vi "mhk_Basic Acquisition_XLS dbl.vi"() -> ()   [LabVIEW 2010]
uses:
  <vilib>/Utility/error.llb/DialogType.ctl
  <vilib>/DAQmx/read.llb/DAQmx Read (Analog 2D DBL NChan NSamp).vi
  <vilib>/DAQmx/create/channels.llb/DAQmx Create Channel (AI-Voltage-Basic).vi
  <vilib>/DAQmx/configure/timing.llb/DAQmx Timing (Sample Clock).vi
  <vilib>/daqmx/miscellaneous.llb/DAQmx Fill In Error Info.vi
  <vilib>/Utility/file.llb/Write To Spreadsheet File (DBL).vi
panel:
  out "# of pts per \nchannel":i32=100
  out "# of channels \nacquired":i32=2
  out "dt (sec)":dbl=0.0001
  in  "Save Data?":bool caption="Enable"
  in  "Maximum Value":dbl=5.0 format="%0.2f"
  in  "Minimum Value":dbl=-5.0 format="%0.2f"
  in  "Physical Channel":tag="Dev2/ai1:2"
  in  "Rate":dbl=10000.0 caption="Sample Rate (Hz)" format="%0.2f"
  in  "Samples per Channel":i32=100
  out "Measurement":cluster{i32, dbl, dbl[][]}(graph)={0, 0.0001, [[0.11978514969328898, 0.31235694448683127, 0.5038605914487136, 0.9799493392742699, 1.3254188665425581, 1.5303506576738792, 1.7484054078798792, 1.9394512771996215, 2.446058534501175, 2.4918362987151705, 2.93603320413831, 2.975402081362346, 3.4054078798791467, 3.576158940397351, 3.8329721976378672, 3.956266975920896, 4.169743949705496, 4.3510238959929195, 4.386120181890316, 4.5689260536515395, 4.546189764091921, 4.728995635853145, 4.6163823358867155, 4.819635608996856, 4.770348216193121, 4.813226722006897, 4.697256385998108, 4.821619312112796, 4.775994140446181, 4.627063814203314, 4.619434186834315, 4.470046082949309, 4.2544328135013885, 4.333475753044222, 4.042023987548448, 3.902401806695761, 3.7987914670247505, 3.4376049073763237, 3.230994598223823, 2.945036164433729, 2.93557542649617, 2.576525162511063, 2.383648182622761, 1.945860164189581, 1.641285439619129, 1.5956602679525131, 1.1384929960020753, 0.9956663716544084, 0.5467390972624897, 0.21317178868984038, 0.07248146000549333, -0.3666798913541063, -0.47242652668843654, -0.8313241981261635, -1.2146366771446881, -1.4604632709738457, -1.717886898403882, -2.0393993957335126, -2.228156376842555, -2.4820703756828517, -2.903378398998993, -3.0289620654927214, -3.4209723197119053, -3.6365855891598255, -3.7022003845332194, -3.8224433118686485, -3.945432905056917, -4.382610553300577, -4.406109805597095, -4.446699423200171, -4.618823816644795, -4.586626789147618, -4.89638966032899, -4.943693350016785, -4.701528977324747, -4.8908963286233105, -4.927671132541887, -4.89410077211829, -4.78408154545732, -4.791405987731559, -4.520554216132084, -4.551377910702842, -4.387188329721976, -4.12991729483932, -4.166997283852656, -3.988616595965453, -3.872493667409284, -3.493301187170019, -3.347880489516892, -2.953886532181768, -2.865840632343516, -2.6267281105990783, -2.461012604144414, -2.0392468031861326, -1.7902157658619953, -1.358073671681875, -1.259956663716544, -0.9611804559465316, -0.511490218817713, -0.3338724936674093], [0.48097170934171574, 0.5813776055177465, 1.0701315347758416, 1.3006988738670002, 1.4848780785546434, 2.024445326090274, 2.28354747154149, 2.377391888180181, 2.8096865749076816, 2.9644154179509874, 3.224433118686483, 3.325296792504654, 3.5700552385021513, 3.7896359141819516, 4.040955839716788, 4.079561754203925, 4.179204687643056, 4.556108279671621, 4.571520126956999, 4.757835627307962, 4.866023743400373, 4.8271126438184755, 4.6812341685232095, 4.770653401287881, 4.831080050050356, 4.752342295602283, 4.935148167363506, 4.6653645435956905, 4.738151188695944, 4.67909787285989, 4.609515671254616, 4.408398693807794, 4.144108401745659, 3.903012176885281, 3.9382610553300577, 3.80230109561449, 3.4612567522202218, 3.3538315988647116, 3.0941190832239753, 2.641224402600177, 2.359080782494583, 2.3191015350810265, 1.8089846491897337, 1.8016602069154943, 1.5018158513138218, 1.2016663106173895, 0.8290353099154637, 0.46800134281441697, 0.12222663045136875, -0.18448438978240303, -0.4924161503952147, -0.6015198217719047, -0.967589342936491, -1.2805566576128422, -1.4664143803216652, -1.7743461409344767, -2.0285653248695334, -2.414471877193518, -2.7007354960783716, -3.0053102206488234, -3.108157597582934, -3.392590105899228, -3.595843379009369, -3.7598803674428543, -3.9182714316232796, -4.154942472609638, -4.303567613757744, -4.400311288796655, -4.573656422620319, -4.791100802636799, -4.645527512436293, -4.832453382976776, -4.792474135563219, -4.920041505172887, -4.7949156163212985, -4.916684469130527, -4.857020783104953, -4.829096346934416, -4.718619342631306, -4.5365764336069825, -4.4392223883785515, -4.475081637012848, -4.183019501327555, -3.9310892056031985, -3.783989989928892, -3.6460463270973844, -3.3169042023987547, -3.087710196234016, -3.055207983642079, -2.687002166814173, -2.5399029511398665, -2.2985015411847285, -1.9431134983367413, -1.6838587603381452, -1.2489700003051851, -1.173741874446852, -0.7335123752555925, -0.5098117007965332, -0.06988738670003357, -0.02075258644367809]]}
  # "Channel Parameters"
  # "Timing Parameters"
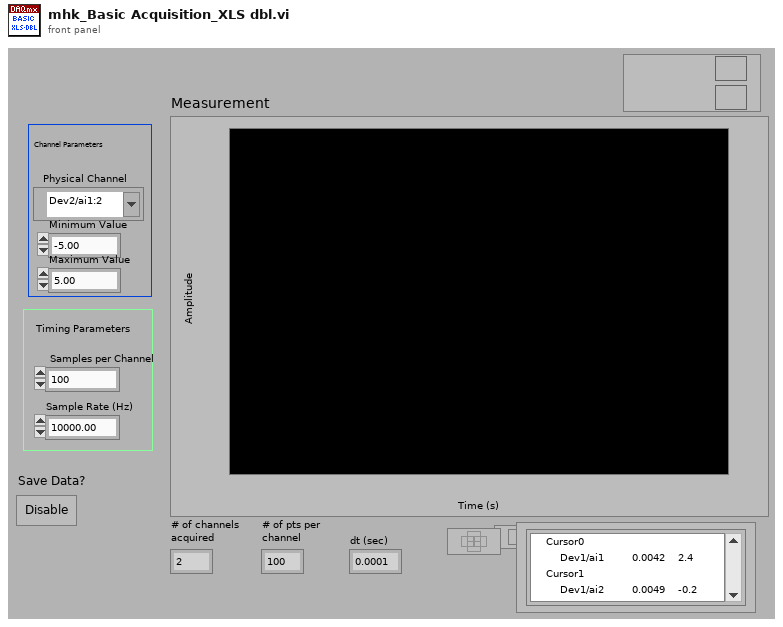
[diagram p1: front panel]
types:
  T1 = typedef "DialogType.ctl" = u16
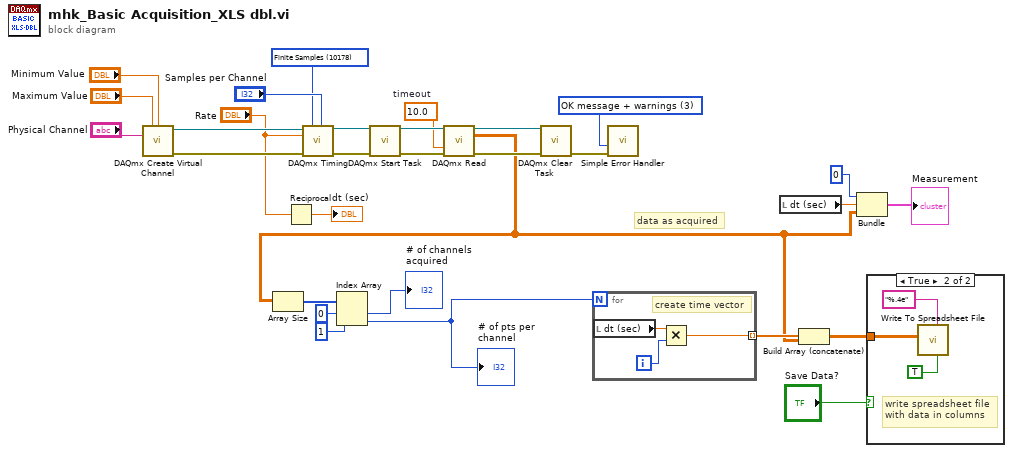
[diagram p0: block diagram]
diagram:
  w15 = T1 3 items=["no dialog", "OK message", "continue or stop message", "OK message + warnings", "continue/stop + warnings"] ("type of dialog (OK msg:1)")
  w16 = 10.0  # timeout
  w20 = 10178 items=["Finite Samples"=10178, "Continuous Samples"=10123] ("sample mode")
  # "data as acquired"
  n1 = call-poly <vilib>:"DAQmx Create Virtual Channel.vi"("maximum value"="Maximum Value", "minimum value"="Minimum Value", "physical channels"="Physical Channel") -> ("task out"=w24:refnum<k21>, "error out"=w28:errorcluster)  [unwired: 11 in]
  n2 = Reciprocal(x="Rate") -> (1/x=→"dt (sec)":dbl)
  n3 = call-poly <vilib>:"DAQmx Timing.vi"("task/channels in"=w24, "sample mode"=w20, "samples per channel"="Samples per Channel", "rate"="Rate", "error in"=w28) -> ("task out"=w19:refnum<k21>, "error out"=w18:errorcluster)  [unwired: 9 in]
  n4 = call <vilib>:"DAQmx Start Task.vi"("task/channels in"=w19, "error in"=w18) -> ("task out"=w23:refnum<k21>, "error out"=w27:errorcluster)  [unwired: 12 in]
  n5 = call-poly <vilib>:"DAQmx Read.vi"("task/channels in"=w23, "timeout"=w16, "error in"=w27) -> ("task out"=w22:refnum<k21>, "data"=w8:dbl[][], "error out"=w17:errorcluster)  [unwired: 10 in]
  n6 = Array Size(array=w8) -> (size(s)=w14:i32[])
  n7 = Index Array(array=w14, index #1=0 ("index"), index #2=1 ("index")) -> (element #1=→"# of channels \nacquired":i32, element #2=w4:i32)
  "# of pts per \nchannel" <- w4
  n8 = call <vilib>:"DAQmx Clear Task.vi"("task in"=w22, "error in"=w17) -> ("error out"=w25:errorcluster)  [unwired: 13 in]
  n9 = for {
    N: w4 -> [_]
    tunnel: [w32] -> w9 mode=indexing
    i -> [w33]
    # "create time vector"
    n10 = local read "dt (sec)"() -> (w31:dbl)
    n11 = Multiply(x=w31, y=w33) -> (x*y=w32:dbl)
  }
  n12 = call <vilib>:"Simple Error Handler.vi"("type of dialog (OK msg:1)"=w15, "error in (no error)"=w25) -> ()  [unwired: 3 in, 5 out]
  n13 = local read "dt (sec)"() -> (w5:dbl)
  n14 = Build Array (concatenate)(w9, w8) -> (w3:dbl[][])
  n15 = Bundle(0, "dt (sec)"=w5, "data"=w8) -> (→"Measurement":cluster{i32, "dt (sec)":dbl, "data":dbl[][]})  [unwired: 1 in]
  n16 = case shown="True" "Save Data?" {
    tunnel: w3 -> [_ w35]
    frame False {
    }
    frame True {
      # "write spreadsheet file\nwith data in columns"
      n17 = call-poly <vilib>:"Write To Spreadsheet File.vi"("transpose? (no:F)"=TRUE, "format (%.3f)"="%.4e", "2D data"=w35) -> ()  [unwired: 5 in, 1 out]
    }
  }
